vi "New Node.vi"(8 "error in (no error)":errorcluster, 10 "UID":string, 11 "UA Server in":refnum<class "UA Server.lvclass">) -> (0 "error out":errorcluster, 2 "Generic Node out":refnum<class "Generic Node.lvclass">, 3 "UA Server out":refnum<class "UA Server.lvclass">)   [LabVIEW 2017, in "Browser Core.lvlib" / "UA Server.lvclass"]
doc: "Create new Node Class from UID Input"
uses:
  UA Server.lvclass
  Node Classes/Generic Node/Generic Node.lvclass
  Node Classes/UA Node/UA Node.lvclass
  C:/Users/MattJ/Desktop/GitHubSCM/UA-Server-Browser/source/Browser Core/Node Classes/Generic Node/Generic Node.lvclass
  Node Classes/UA Node/Node Class.ctl
  UA Server.lvclass/UA Server.ctl
  Node Classes/Generic Node/Generic Node.lvclass/Generic Node.ctl
  Node Classes/UA Node/UA Node.lvclass/UA Node.ctl
  <vilib>/OPCUA/NI OPC UA Client.lvlib
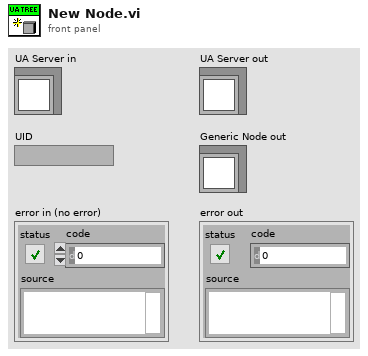
[diagram p1: front panel]
types:
  T1 = typedef "Browser Core.lvlib/UA Node.lvclass/Node Class.ctl" = u16
  T2 = typedef "OPC UA Client Refnum.ctl" = refnum<k21>
  T3 = typedef "Data Type Indicator.ctl" = u16
  T4 = cluster{"name":string, "node class":u16, "data type":T3, "access":enum16{"Null", "Read", "Write", "Read&Write"}, "description":string}
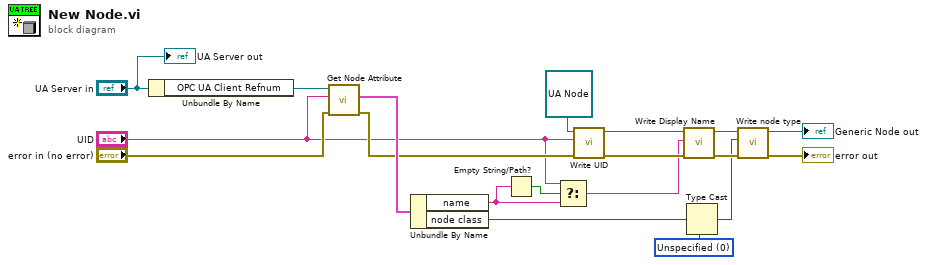
[diagram p0: block diagram]
diagram:
  w7 = T1 0 items=["Unspecified"=0, "Object"=1, "Variable"=2, "Method"=4, "Object Type"=8, "Variable Type"=16, "Reference Type"=32, "Data Type"=64, "View"=128] ("node class")
  n1 = Unbundle By Name("UA Server in") -> ("OPC UA Client Refnum"=w19:T2)
  n2 = call <vilib>:"Get Node Attribute.vi"("error in (no error)"="error in (no error)", "node ID"="UID", "OPC UA client refnum in"=w19) -> ("error out"=w5:errorcluster, "node attribute"=w17:T4)  [unwired: 5 in, 2 out]
  n3 = Unbundle By Name(w17) -> ("name"=w2:string, "node class"=w9:u16)
  n4 = Empty String/Path?(string/path=w2) -> (empty?=w4:bool)
  n5 = Select(t="UID", s=w4, f=w2) -> (s? t:f=w1:string)
  n6 = call "Write UID.vi"("error in (no error)"=w5, "UID"="UID", "Generic Node in"=refnum<class "UA Node.lvclass"> refnum ("Browser Core.lvlib:UA Node.lvclass")) -> ("error out"=w15:errorcluster, "Generic Node out"=w16:refnum<class "UA Node.lvclass">)  [unwired: 7 in]
  n7 = call "Write Display Name.vi"("error in (no error)"=w15, "Display Name"=w1, "Generic Node in"=w16) -> ("error out"=w13:errorcluster, "Generic Node out"=w14:refnum<class "UA Node.lvclass">)  [unwired: 7 in]
  n8 = Type Cast(type=w7, x=w9) -> (*(type *) &x=w8:T1)
  n9 = call "Write node type.vi"("error in (no error)"=w13, "node class"=w8, "UA Node in"=w14) -> ("error out"=→"error out":errorcluster, "UA Node out"=→"Generic Node out":refnum<class "UA Node.lvclass">)  [unwired: 7 in]
  "UA Server out" <- "UA Server in"
